vi "Amium AK Befehl mit Informationen.vi"(10 "AK Befehl":string) -> (2 "String für schreiben":string)   [LabVIEW 2020, in "Amium PNS.lvlib" / "AK Kommunikation.lvlib"]
uses:
  AK Kommunikation.lvlib
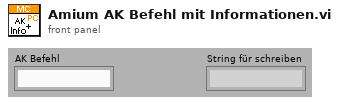
[diagram p1: front panel]
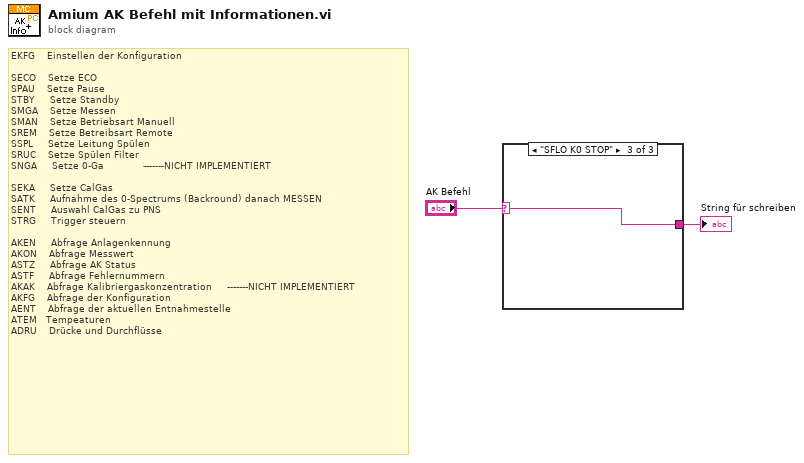
[diagram p0: block diagram]
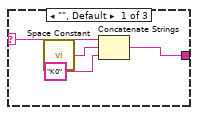
[diagram p2: hidden frame]
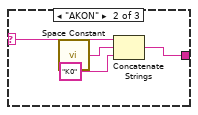
[diagram p3: hidden frame]
diagram:
  # "EKFG    Einstellen der Konfiguration\n\nSECO    Setze ECO\nSPAU    Setze Pause\nSTBY     Setze Standby\nSMGA    Setze Messen\nSMAN    Setze Betriebsart Manuell\nSREM    Setze Betreibsart Remote\nSSPL     Setze Leitung Spülen\nSRUC    Setze Spülen Filter\nSNGA     Setze 0-Ga             -------NICHT IMPLEMENTIERT\n\nSEKA     Setze CalGas\nSATK     Aufnahme des 0-Spectrums (Backround) danach MESSEN\nSENT     Auswahl CalGas zu PNS\nSTRG     Trigger steuern\n\nAKEN     Abfrage Anlagenkennung\nAKON    Abfrage Messwert\nASTZ     Abfrage AK Status\nASTF     Abfrage Fehlernummern\nAKAK    Abfrage Kalibriergaskonzentration     -------NICHT IMPLEMENTIERT\nAKFG    Abfrage der Konfiguration\nAENT    Abfrage der aktuellen Entnahmestelle\nATEM   Tempeaturen\nADRU    Drücke und Durchflüsse"
  n1 = case shown="\"SFLO K0 STOP\"" "AK Befehl" {
    selector: "AK Befehl" -> [w4 w10 w11]
    tunnel: [w3 w7 w11] -> w2
    frame "", Default {
      n2 = call <vilib>:"Space Constant.vi"() -> ("String"=w6:string)
      n3 = Concatenate Strings(w4, w6, "K0" ("String")) -> (w3:string)
    }
    frame "AKON" {
      n4 = call <vilib>:"Space Constant.vi"() -> ("String"=w9:string)
      n5 = Concatenate Strings(w10, w9, "K0" ("String")) -> (w7:string)
    }
    frame "SFLO K0 STOP" {
    }
  }
  "String für schreiben" <- w2
